vi "Data Point.vi"(7 "Data Point - Cmd":T5, 8 "error in":errorcluster, 11 "Data":variant) -> (0 "error out":errorcluster, 3 "Line protocol":string="mem3,host=host1 Temp3=25.43297108\nmem3,host=host1 Temp3=20.79402671\nmem3,host=host1 Temp3=24.95297822\nmem3,host=host1 Temp3=20.65259873\nmem3,host=host1 Temp3=20.9054627\nmem3,host=host1 Temp3=27.02653303\nmem3,host=host1 Temp3=22.08146195\nmem3,host=host1 Temp3=24.19398422\nmem3,host=host1 Temp3=19.31873737\nmem3,host=host1 Temp3=20.74735395\nmem3,host=host1 Temp3=23.15595401\nmem3,host=host1 Temp3=24.42632595\nmem3,host=host1 Temp3=28.3766217\nmem3,host=host1 Temp3=19.89789073\nmem3,host=host1 Temp3=26.53353835\nmem3,host=host1 Temp3=23.88864325\nmem3,host=host1 Temp3=27.71056479\nmem3,host=host1 Temp3=21.0755503\nmem3,host=host1 Temp3=19.07104004\nmem3,host=host1 Temp3=20.45387692\nmem3,host=host1 Temp3=19.72276944\nmem3,host=host1 Temp3=22.96587107\nmem3,host=host1 Temp3=25.03849142\nmem3,host=host1 Temp3=25.11178574\nmem3,host=host1 Temp3=20.4397148\nmem3,host=host1 Temp3=23.22899956\nmem3,host=host1 Temp3=22.09242219")   [LabVIEW 2020, in "InfluxDB v2 Client.lvlib"]
uses:
  InfluxDB v2 Client.lvlib
  Data Point - Cmd.ctl
  Data Point.ctl
  Tag.ctl
  Field.ctl
  Timestamp precision.ctl
panel:
  out "Data Point":T1 {"Time Stamp" format="%<%x %.3X>T"}
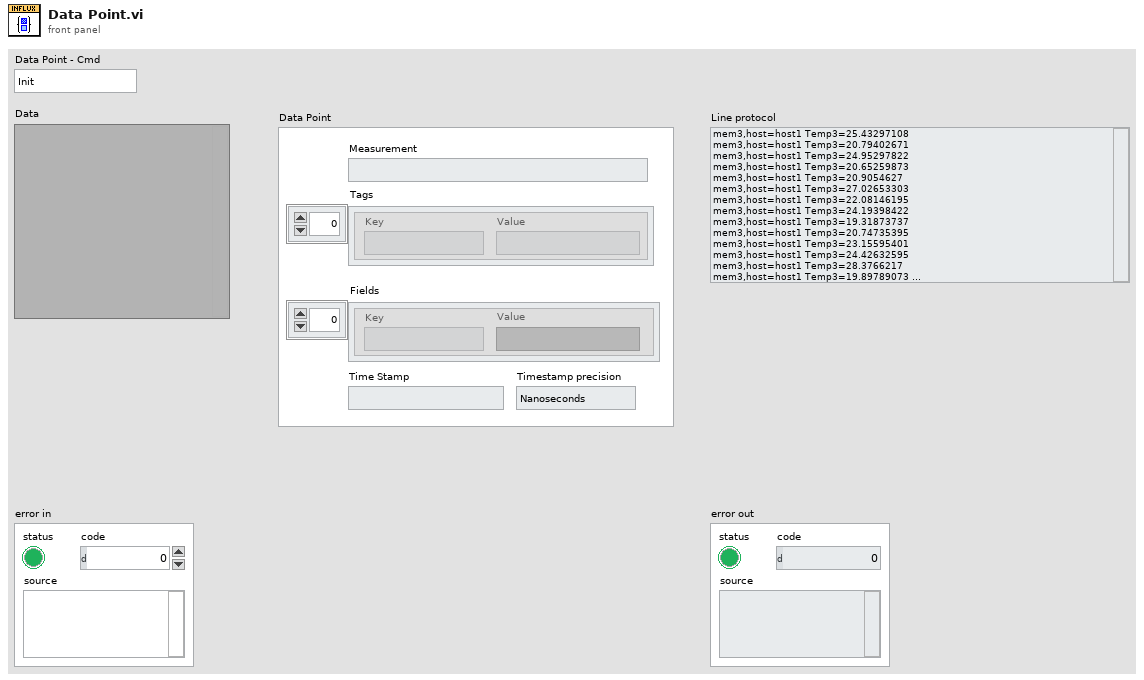
[diagram p1: front panel]
types:
  T1 = typedef "InfluxDB v2 Client.lvlib/Data Point.ctl" = cluster{"Measurement":string, "Tags":T2[], "Fields":T3[], "Timestamp precision":T4, "Time Stamp":timestamp}
  T2 = typedef "InfluxDB v2 Client.lvlib/Tag.ctl" = cluster{"Key":string, "Value":string}
  T3 = typedef "InfluxDB v2 Client.lvlib/Field.ctl" = cluster{"Key":string, "Value":variant}
  T4 = typedef "InfluxDB v2 Client.lvlib/Timestamp precision.ctl" = enum16{"Nanoseconds", "Microseconds", "Milliseconds", "Seconds"}
  T5 = typedef "InfluxDB v2 Client.lvlib/Data Point - Cmd.ctl" = enum16{"Init", "Add Tags", "Add Fields", "Add Field Names", "Add Field Values", "Add Measurement", "Add Time Stamp", "Add Precision", "Get Line Protocol"}
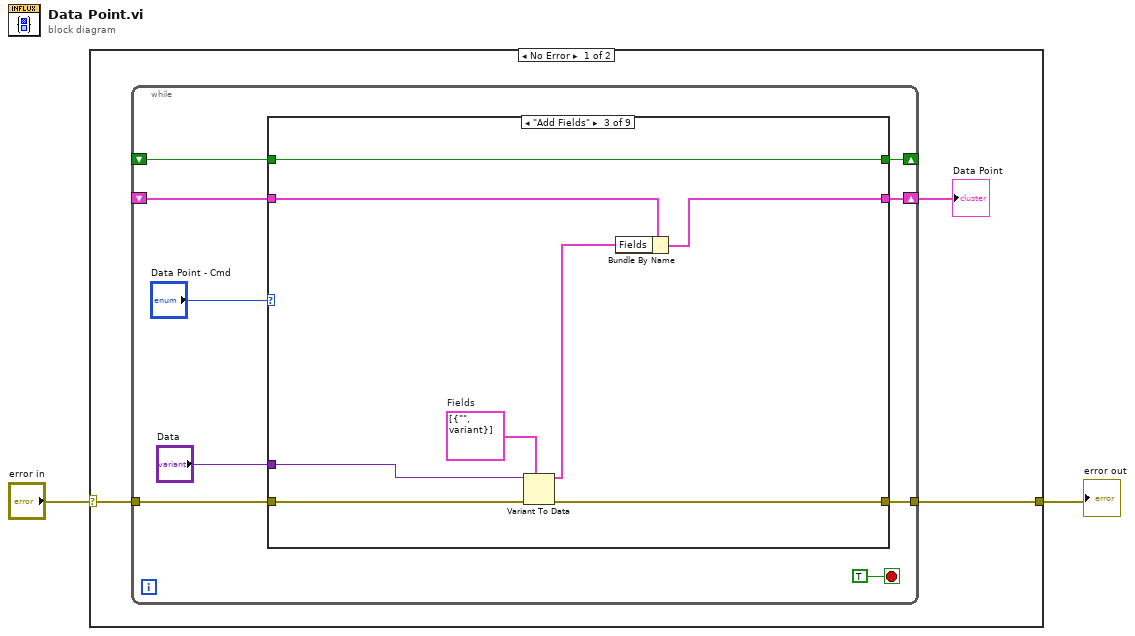
[diagram p0: block diagram]
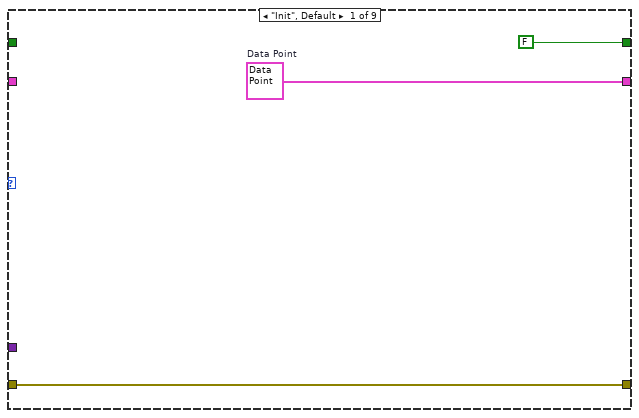
[diagram p2: hidden frame]
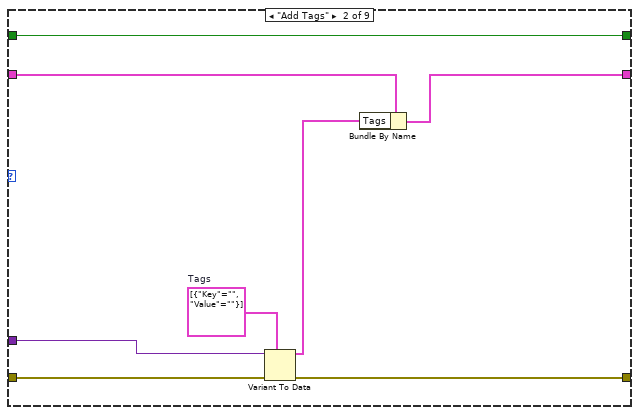
[diagram p3: hidden frame]
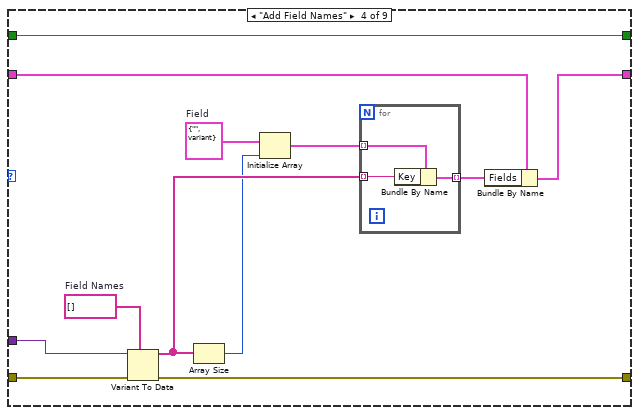
[diagram p4: hidden frame]
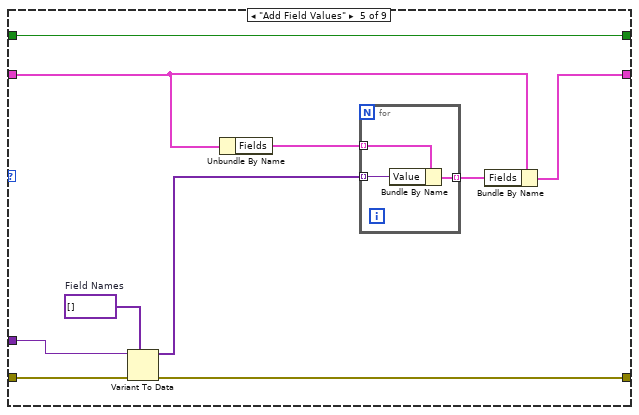
[diagram p5: hidden frame]
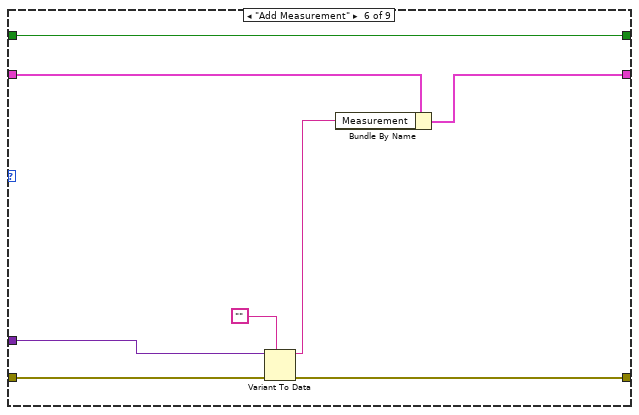
[diagram p6: hidden frame]
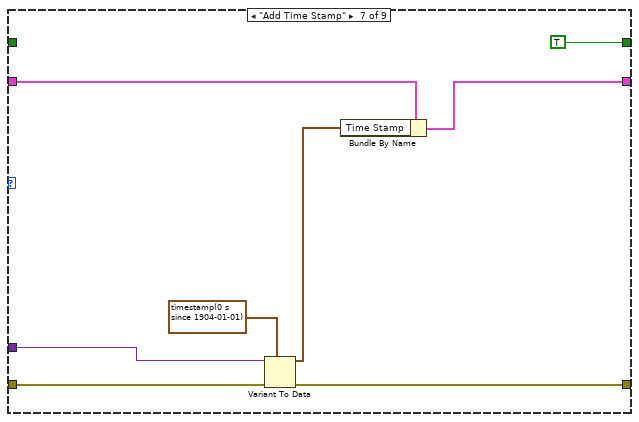
[diagram p7: hidden frame]
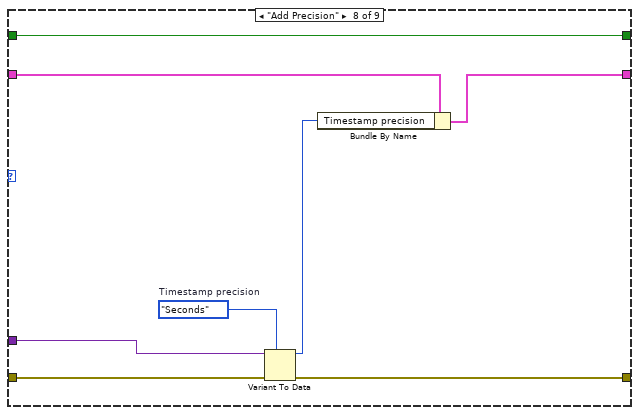
[diagram p8: hidden frame]
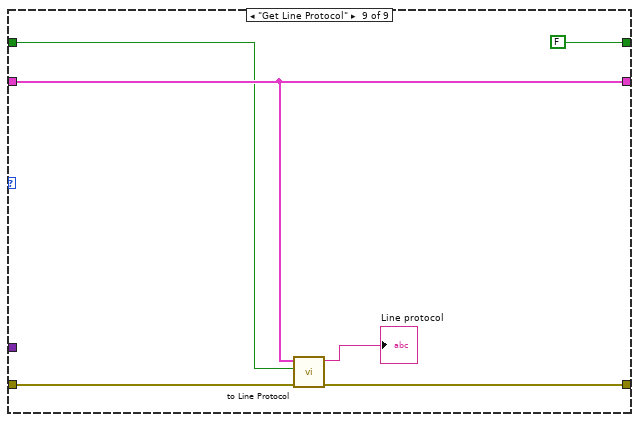
[diagram p9: hidden frame]
diagram:
  n1 = case shown="No Error" "error in" {
    selector: "error in" -> [w5 w92]
    tunnel: [w4 w92] -> w1
    frame No Error {
      n2 = while {
        tunnel: w5 -> [w12]
        tunnel: [w11] -> w4
        shift-right: [w10] -> w3
        shift-left: _ -> [w9]
        shift-right: [w7] -> _
        shift-left: _ -> [w6]
        stop <- TRUE stop-if-true
        n3 = case shown="\"Add Fields\"" "Data Point - Cmd" {
          tunnel: w12 -> [w17 w25 w33 w45 w58 w69 w77 w85 w91]
          tunnel: [w17 w24 w32 w44 w57 w68 w76 w84 w90] -> w11
          tunnel: [w16 w20 w28 w42 w55 w65 w73 w81 w88] -> w10
          tunnel: w9 -> [_ w21 w29 w40 w50 w66 w74 w82 w88]
          tunnel: "Data" -> [_ w23 w31 w43 w56 w67 w75 w83 _]
          tunnel: [FALSE w18 w26 w41 w54 w62 TRUE w78 FALSE] -> w7
          tunnel: w6 -> [_ w18 w26 w41 w54 w62 _ w78 w87]
          frame "Init", Default {
            w16 = T1 {"Measurement"="", "Tags"=[], "Fields"=[], "Timestamp precision"=enum."Nanoseconds", "Time Stamp"=timestamp(0 s since 1904-01-01)}  # Data Point
          }
          frame "Add Tags" {
            w22 = T2[] [{"Key"="", "Value"=""}]  # Tags
            n4 = Variant To Data(error in=w25, type=w22, Variant=w23) -> (data=w19:T2[], error out=w24:errorcluster)
            n5 = Bundle By Name(cluster=w21, "Tags"=w19) -> (w20:T1)
          }
          frame "Add Fields" {
            w30 = T3[] [{"Key"="", "Value"=variant}]  # Fields
            n6 = Variant To Data(error in=w33, type=w30, Variant=w31) -> (data=w27:T3[], error out=w32:errorcluster)
            n7 = Bundle By Name(cluster=w29, "Fields"=w27) -> (w28:T1)
          }
          frame "Add Field Names" {
            w36 = T3 {"Key"="", "Value"=variant}  # Field
            w37 = string[] []  # Field Names
            n8 = Variant To Data(error in=w45, type=w37, Variant=w43) -> (data=w39:string[], error out=w44:errorcluster)
            n9 = Array Size(array=w39) -> (size(s)=w38:i32)
            n10 = Initialize Array(w36, w38) -> (w35:T3[])
            n11 = for {
              tunnel: w39 -> [w46] mode=indexing
              tunnel: [w48] -> w34 mode=indexing
              tunnel: w35 -> [w47] mode=indexing
              n12 = Bundle By Name(cluster=w47, "Key"=w46) -> (w48:T3)
            }
            n13 = Bundle By Name(cluster=w40, "Fields"=w34) -> (w42:T1)
          }
          frame "Add Field Values" {
            w52 = variant[] []  # Field Names
            n14 = Variant To Data(error in=w58, type=w52, Variant=w56) -> (data=w53:variant[], error out=w57:errorcluster)
            n15 = Unbundle By Name(w50) -> ("Fields"=w49:T3[])
            n16 = for {
              tunnel: w53 -> [w59] mode=indexing
              tunnel: [w61] -> w51 mode=indexing
              tunnel: w49 -> [w60] mode=indexing
              n17 = Bundle By Name(cluster=w60, "Value"=w59) -> (w61:T3)
            }
            n18 = Bundle By Name(cluster=w50, "Fields"=w51) -> (w55:T1)
          }
          frame "Add Measurement" {
            n19 = Variant To Data(error in=w69, type="", Variant=w67) -> (data=w64:string, error out=w68:errorcluster)
            n20 = Bundle By Name(cluster=w66, "Measurement"=w64) -> (w65:T1)
          }
          frame "Add Time Stamp" {
            n21 = Variant To Data(error in=w77, type=timestamp(0 s since 1904-01-01), Variant=w75) -> (data=w72:timestamp, error out=w76:errorcluster)
            n22 = Bundle By Name(cluster=w74, "Time Stamp"=w72) -> (w73:T1)
          }
          frame "Add Precision" {
            w79 = Timestamp_precision."Seconds"  # Timestamp precision
            n23 = Variant To Data(error in=w85, type=w79, Variant=w83) -> (data=w80:T4, error out=w84:errorcluster)
            n24 = Bundle By Name(cluster=w82, "Timestamp precision"=w80) -> (w81:T1)
          }
          frame "Get Line Protocol" {
            n25 = call "to Line Protocol.vi"("error in"=w91, "Use Timestamp?"=w87, "Data Point"=w88) -> ("error out"=w90:errorcluster, "Line Protocol"=→"Line protocol":string)  [unwired: 7 in]
          }
        }
      }
      "Data Point" <- w3
    }
    frame Error {
    }
  }
  "error out" <- w1
